vi "Load Settings from XML.vi"(8 "error in (no error)":errorcluster, 11 "Settings in":T1={"Hardware Configuration"={"DAQmx Channel"="cDAQETH/ai0:23, cDAQETH/ai29, cDAQETH/ai31:30", "Sample Rate"=1000.0, "DAQmx Task"="", "ResetInterp"=FALSE, "GainConstants"=[0.01, 2.0, 10.0, 1.0, 0.1], "FilterCoefficients"=[[1.0], [1.0]], "ChannelNames"=["CH1X", "CH1Y", "CH1Z", "CH2X", "CH2Y", "CH2Z", "CH3X", "CH3Y", "CH3Z", "CH4X", "CH4Y", "CH4Z", "CH5X", "CH5Y", "CH5Z", "CH6X", "CH6Y", "CH6Z", "CH7X", "CH7Y", "CH7Z", "CH8X", "CH8Y", "CH8Z"], "ActiveChannels"=[], "Display Rate"=0, "ResponseExtension"=TRUE}, "Logging Configuration"={"Log File Base Path"=path "D:/Documents/LabVIEW Data/Logged Data.tdms", "Samples to Save"=9900, "Trigger - Threshold"=0.0, "Trigger - Channel"=0, "Always Log"=FALSE, "External Trigger"=TRUE, "External Trigger Armed"=FALSE, "TDMS File Reference"=refnum, "DAQVersion"="1.0", "SWVersion"="1.7.5.12", "CircSamples"=100, "BeepWhenComplete"=TRUE, "ChannelConfig"=[["CH1", "CH1", "NA", "XYZ"], ["CH2", "CH2", "NA", "XYZ"], ["CH3", "CH3", "NA", "XYZ"], ["CH4", "CH4", "NA", "XYZ"], ["CH5", "CH5", "NA", "XYZ"], ["CH6", "CH6", "NA", "XYZ"], ["CH7", "CH7", "NA", "XYZ"], ["CH8", "CH8", "NA", "XYZ"]], "ActiveChannels"=[], "Title"="Title", "Description"="Description....", "ChannelNames"=["CH1X", "CH1Y", "CH1Z", "CH2X", "CH2Y", "CH2Z", "CH3X", "CH3Y", "CH3Z", "CH4X", "CH4Y", "CH4Z", "CH5X", "CH5Y", "CH5Z", "CH6X", "CH6Y", "CH6Z", "CH7X", "CH7Y", "CH7Z", "CH8X", "CH8Y", "CH8Z"], "ResponseExtension"=TRUE}}) -> (0 "error out":errorcluster, 3 "Settings out":T1={"Hardware Configuration"={"DAQmx Channel"="", "Sample Rate"=0.0, "DAQmx Task"="", "ResetInterp"=FALSE, "GainConstants"=[], "FilterCoefficients"=[], "ChannelNames"=[], "ActiveChannels"=[], "Display Rate"=1000, "ResponseExtension"=TRUE}, "Logging Configuration"={"Log File Base Path"=path "", "Samples to Save"=0, "Trigger - Threshold"=0.0, "Trigger - Channel"=0, "Always Log"=FALSE, "External Trigger"=FALSE, "External Trigger Armed"=FALSE, "TDMS File Reference"=refnum, "DAQVersion"="", "SWVersion"="", "CircSamples"=0, "BeepWhenComplete"=FALSE, "ChannelConfig"=[], "ActiveChannels"=[], "Title"="", "Description"="", "ChannelNames"=[], "ResponseExtension"=TRUE}})   [LabVIEW 2017, in "Settings.lvlib"]
doc: "Attempts to load previous user specified settings from an XML file.\n\nThis VI will not generate an error. If a suitable XML file can't be loaded and parsed then it will simply return the default settings."
uses:
  Settings.lvlib
  Settings.ctl
  Acquisition/Hardware Configuration.ctl
  Logging/Logging Configuration.ctl
  <vilib>/Utility/file.llb/Read Delimited Spreadsheet (DBL).vi
  <vilib>/Utility/xml.llb/Read From XML File(string).vi
  <vilib>/Utility/xml.llb/Write to XML File(string).vi
  <resource>/objmgr/daqmx.rc
  Acquisition/Acquisition.lvlib
  Logging/Logging.lvlib
panel:
  # "(Scroll up for Settings Controls)"
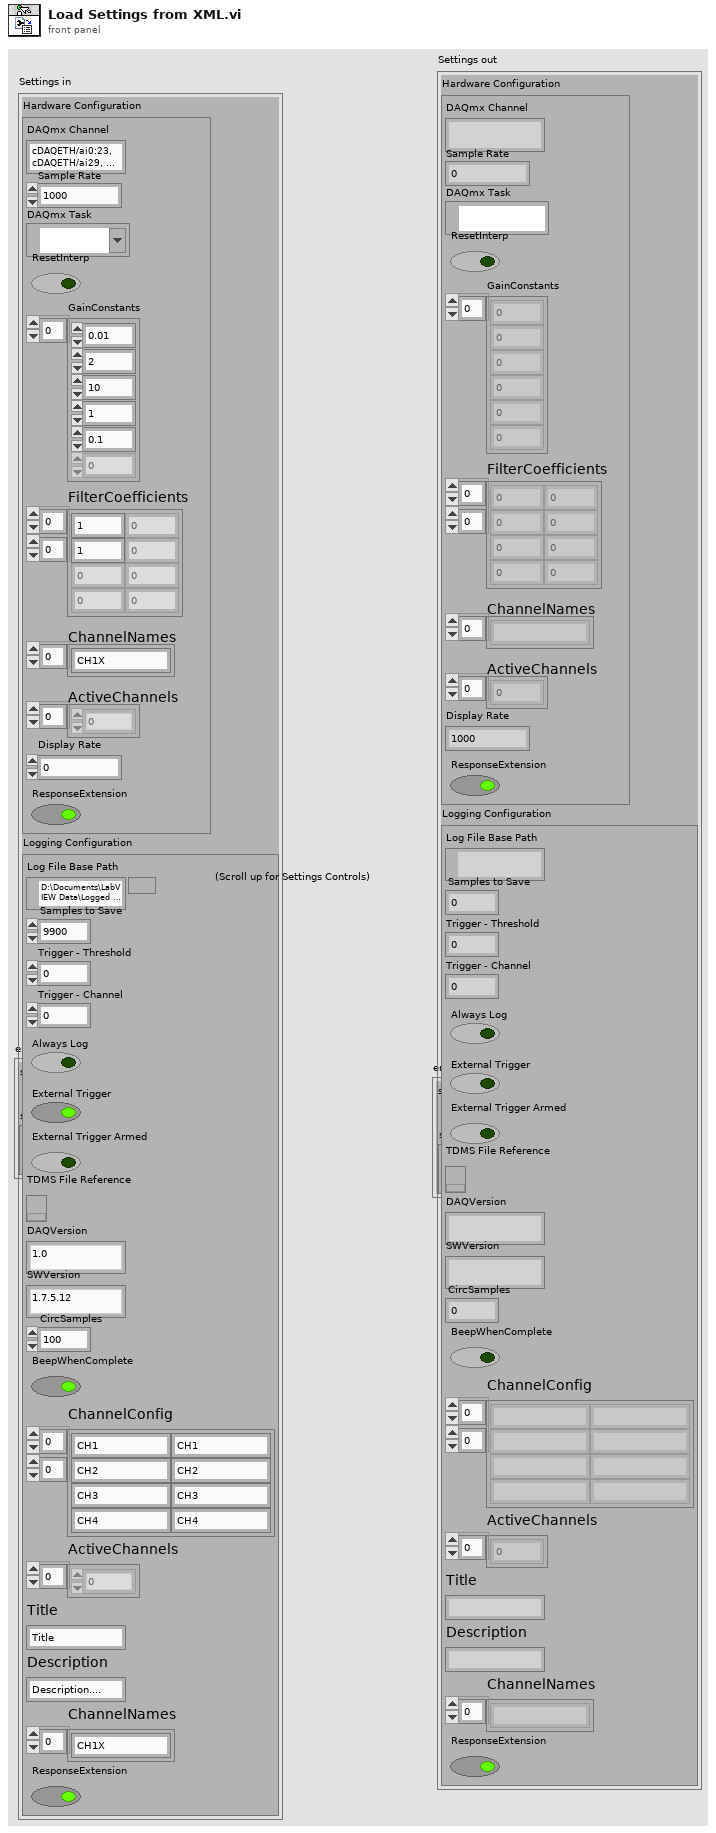
[diagram p1: front panel]
types:
  T1 = typedef "Settings.lvlib/Settings.ctl" = cluster{"Hardware Configuration":T2, "Logging Configuration":T3}
  T2 = typedef "Acquisition.lvlib/Hardware Configuration.ctl" = cluster{"DAQmx Channel":string, "Sample Rate":dbl, "DAQmx Task":refnum<k21>, "ResetInterp":bool, "GainConstants":dbl[], "FilterCoefficients":dbl[][], "ChannelNames":string[], "ActiveChannels":i32[], "Display Rate":i32, "ResponseExtension":bool}
  T3 = typedef "Logging.lvlib/Logging Configuration.ctl" = cluster{"Log File Base Path":path, "Samples to Save":u32, "Trigger - Threshold":dbl, "Trigger - Channel":u32, "Always Log":bool, "External Trigger":bool, "External Trigger Armed":bool, "TDMS File Reference":refnum<k34>, "DAQVersion":string, "SWVersion":string, "CircSamples":u32, "BeepWhenComplete":bool, "ChannelConfig":string[][], "ActiveChannels":i32[], "Title":string, "Description":string, "ChannelNames":string[], "ResponseExtension":bool}
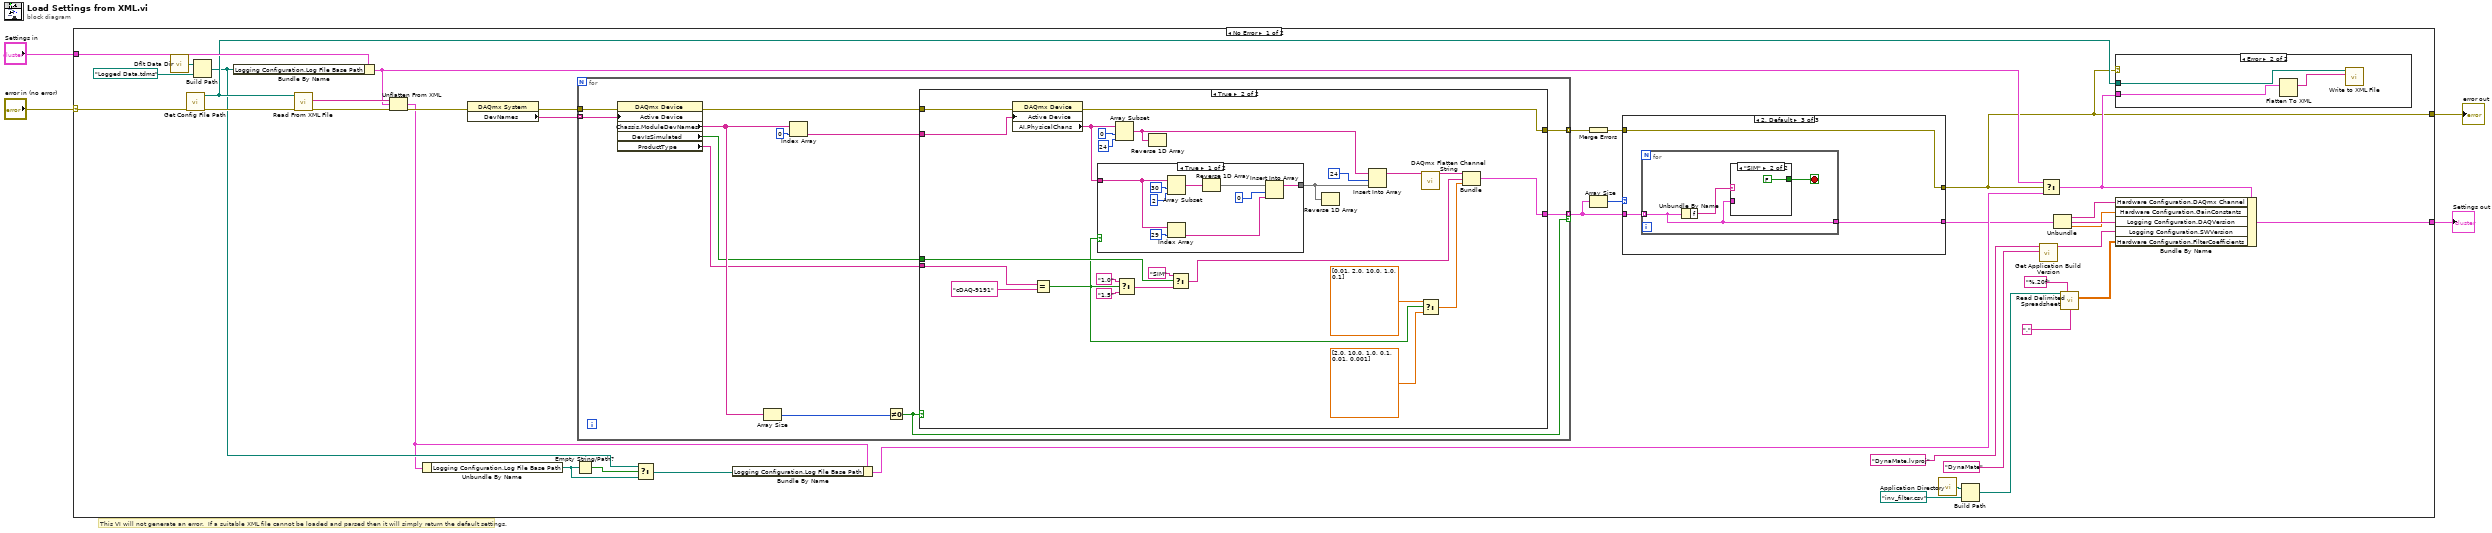
[diagram p0: block diagram]
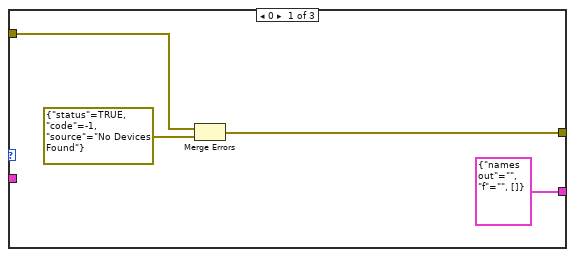
[diagram p2: hidden frame]
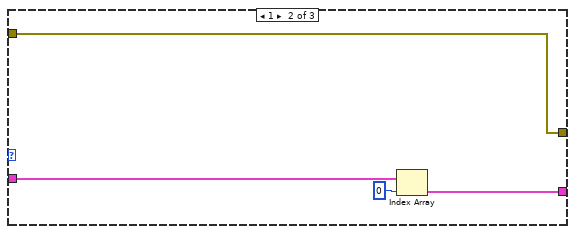
[diagram p3: hidden frame]
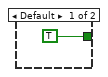
[diagram p4: hidden frame]
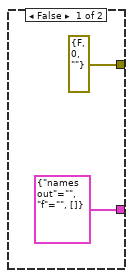
[diagram p5: hidden frame]
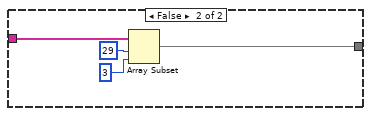
[diagram p6: hidden frame]
diagram:
  # "This VI will not generate an error.  If a suitable XML file cannot be loaded and parsed then it will simply return the default settings."
  n1 = case shown="No Error" "error in (no error)" {
    selector: "error in (no error)" -> [w40 w114]
    tunnel: [w5 w114] -> w3
    tunnel: "Settings in" -> [w39 w113]
    tunnel: [w26 w113] -> w1
    frame No Error {
      n2 = call <vilib>:"Dflt Data Dir.vi"() -> ("App:Default Data Directory"=w38:path)
      n3 = call "Get Config File Path.vi"("error in (no error)"=w40) -> ("error out"=w42:errorcluster, "XML File Path"=w36:path)  [unwired: 9 in]
      n4 = Build Path(base path=w38, name or relative path=path "Logged Data.tdms" ("App:Default Data Directory")) -> (appended path=w30:path)
      n5 = Bundle By Name(cluster=w39, "Logging Configuration.Log File Base Path"=w30) -> (w15:T1)
      n6 = call-poly <vilib>:"Read From XML File.vi"("error in (no error)"=w42, "XML File Path"=w36) -> ("error out"=w35:errorcluster, "XML Elements"=w41:string)  [unwired: 7 in, 1 out]
      n7 = Unflatten From XML(xml string=w41, type=w15, error in (no error)=w35) -> (value=w27:T1, error out=w28:errorcluster)
      n8 = Unbundle By Name(w27) -> ("Logging Configuration.Log File Base Path"=w31:path)
      n9 = property class="DAQmx System"(error in=w28) -> (error out=w14:errorcluster, "DevNames"=w29:tag[])  [unwired: 1 in, 1 out]
      n10 = Empty String/Path?(string/path=w31) -> (empty?=w34:bool)
      n11 = for {
        tunnel: w29 -> [w70] mode=indexing
        tunnel: w14 -> [w69]
        tunnel: [w64] -> w13 mode=indexing
        tunnel: [w60] -> w11 mode=indexing if=w59
        n12 = property class="DAQmx Device"(error in=w69, "Active Device"=w70) -> (error out=w65:errorcluster, "Chassis.ModuleDevNames"=w67:tag[], "DevIsSimulated"=w62:bool, "ProductType"=w61:string)  [unwired: 1 in, 1 out]
        n13 = Array Size(array=w67) -> (size(s)=w68:i32)
        n14 = Index Array(array=w67, index=0) -> (element=w63:tag)
        n15 = Not Equal To 0?(x=w68) -> (x != 0?=w59:bool)
        n16 = case shown="True" w59 {
          tunnel: w65 -> [_ w96]
          tunnel: [errorcluster {"status"=FALSE, "code"=0, "source"=""} ("error out") w95] -> w64
          tunnel: [cluster{"names out":string, "f":string, dbl[]} {"names out"="", "f"="", []} w75] -> w60
          tunnel: w63 -> [_ w90]
          tunnel: w62 -> [_ w86]
          tunnel: w61 -> [_ w81]
          frame False {
          }
          frame True {
            n17 = property class="DAQmx Device"(error in=w96, "Active Device"=w90) -> (error out=w95:errorcluster, "AI.PhysicalChans"=w92:tag[])  [unwired: 1 in, 1 out]
            n18 = Equal?(x=w81, y="cDAQ-9191" ("element")) -> (x = y?=w80:bool)
            n19 = case shown="True" w80 {
              tunnel: w92 -> [w105 w109]
              tunnel: [w99 w106] -> w73
              frame True {
                n20 = Array Subset(array=w105, index=30, length=2) -> (w98:tag[])
                n21 = Index Array(array=w105, index=29) -> (element=w100:tag)
                n22 = Reverse 1D Array(array=w98) -> (reversed array=w97:tag[])
                n23 = Insert Into Array(array=w97, index=0, new element=w100) -> (w99:tag[])
              }
              frame False {
                n24 = Array Subset(array=w109, index=29, length=3) -> (w106:tag[])
              }
            }
            n25 = Array Subset(array=w92, index=0, length=24 ("index")) -> (w74:tag[])
            n26 = Select(t="1.0" ("f"), s=w80, f="1.5") -> (s? t:f=w87:string)
            n27 = Reverse 1D Array(array=w74) -> ()  [unwired: 1 out]
            n28 = Select(t="SIM", s=w86, f=w87) -> (s? t:f=w79:string)
            n29 = Reverse 1D Array(array=w73) -> ()  [unwired: 1 out]
            n30 = Insert Into Array(array=w74, index=24, new element=w73) -> (w77:tag[])
            n31 = call <vilib>:"DAQmx Flatten Channel String.vi"("names in"=w77) -> ("names out"=w76:string)  [unwired: 13 in, 1 out]
            n32 = Select(t=dbl[] [0.01, 2.0, 10.0, 1.0, 0.1], s=w80, f=dbl[] [2.0, 10.0, 1.0, 0.1, 0.01, 0.001]) -> (s? t:f=w78:dbl[])
            n33 = Bundle("names out"=w76, "f"=w79, w78) -> (w75:cluster{"names out":string, "f":string, dbl[]})  [unwired: 1 in]
          }
        }
      }
      n34 = Select(t=w30, s=w34, f=w31) -> (s? t:f=w33:path)
      n35 = Bundle By Name(cluster=w27, "Logging Configuration.Log File Base Path"=w33) -> (w32:T1)
      n36 = Merge Errors(w13) -> (w6:errorcluster)
      n37 = Array Size(array=w11) -> (size(s)=w12:i32)
      n38 = case shown="2, Default" w12 {
        tunnel: w11 -> [_ w49 w53]
        tunnel: [cluster{"names out":string, "f":string, dbl[]} {"names out"="", "f"="", []} w48 w52] -> w10
        tunnel: w6 -> [w43 w47 w51]
        tunnel: [w44 w47 w51] -> w5
        frame 0 {
          n39 = Merge Errors(w43, errorcluster {"status"=TRUE, "code"=-1, "source"="No Devices Found"} ("error IO")) -> (w44:errorcluster)
        }
        frame 1 {
          n40 = Index Array(array=w49, index=0) -> (element=w48:cluster{"names out":string, "f":string, dbl[]})
        }
        frame 2, Default {
          n41 = for {
            tunnel: w53 -> [w55] mode=indexing
            tunnel: [w55] -> w52
            stop <- w54 stop-if-true
            n42 = Unbundle By Name(w55) -> ("f"=w56:string)
            n43 = case shown="\"SIM\"" w56 {
              tunnel: w55 -> [_ _]
              tunnel: [TRUE FALSE] -> w54
              frame Default {
              }
              frame "SIM" {
              }
            }
          }
        }
      }
      n44 = call <vilib>:"Application Directory.vi"() -> ("Application Directory"=w17:path)
      n45 = Build Path(base path=w17, name or relative path=path "inv_filter.csv" ("file path (dialog if empty)")) -> (appended path=w16:path)
      n46 = call "Get Application Build Version.vi"("Build Specification Name"="DynaMate", "Project Filename"="DynaMate.lvproj") -> ("Version String"=w22:string)  [unwired: 7 in, 2 out]
      n47 = Select(t=w15, s=w5, f=w32) -> (s? t:f=w25:T1)
      n48 = Unbundle(w10) -> ("names out"=w9:string, "f"=w8:string, w7:dbl[])
      n49 = call-poly <vilib>:"Read Delimited Spreadsheet.vi"("file path (dialog if empty)"=w16, "format (%.3f)"="%.20f", "delimiter (\\t)"="," ("delimiter (\\t)")) -> ("all rows"=w19:dbl[][])  [unwired: 7 in, 5 out]
      n50 = case shown="Error" w5 {
        tunnel: w25 -> [_ w112]
        tunnel: w36 -> [_ w110]
        frame No Error {
        }
        frame Error {
          n51 = Flatten To XML(anything=w112) -> (xml string=w111:string)
          n52 = call-poly <vilib>:"Write to XML File.vi"("XML Input"=w111, "XML File Path"=w110) -> ()  [unwired: 7 in, 3 out]
        }
      }
      n53 = Bundle By Name(cluster=w25, "Hardware Configuration.DAQmx Channel"=w9, "Hardware Configuration.GainConstants"=w7, "Logging Configuration.DAQVersion"=w8, "Logging Configuration.SWVersion"=w22, "Hardware Configuration.FilterCoefficients"=w19) -> (w26:T1)
    }
    frame Error {
    }
  }
  "error out" <- w3
  "Settings out" <- w1
